vi "Write Array.vi"(8 "error in (no error)":errorcluster, 10 "Array":dbl[](array[numeric]), 11 "Doublo Array in":refnum<class "Doublo Array.lvclass">) -> (0 "error out":errorcluster, 3 "Doublo Array out":refnum<class "Doublo Array.lvclass">)   [LabVIEW 2020, in "Example Source.lvlib" / "Doublo Array.lvclass"]
uses:
  Doublo Array.lvclass
  Doublo Array.lvclass/Doublo Array.ctl
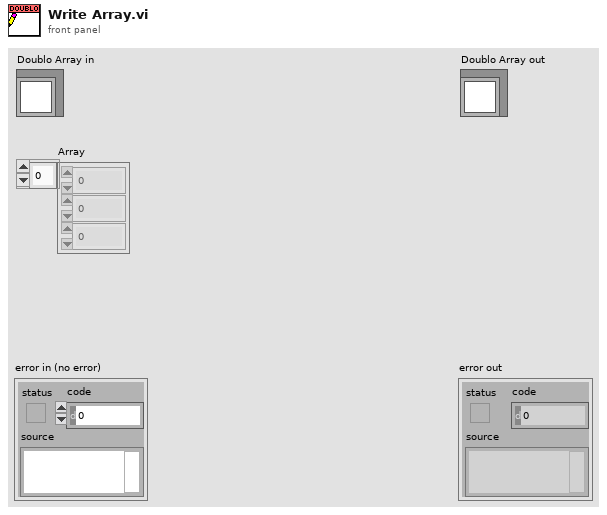
[diagram p1: front panel]
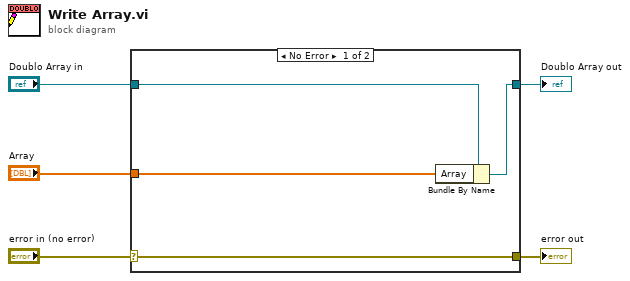
[diagram p0: block diagram]
diagram:
  n1 = case shown="No Error" "error in (no error)" {
    selector: "error in (no error)" -> [w9 w10]
    tunnel: [w9 w10] -> w4
    tunnel: [w7 w11] -> w2
    tunnel: "Doublo Array in" -> [w8 w11]
    tunnel: "Array" -> [w6 _]
    frame No Error {
      n2 = Bundle By Name(cluster=w8, "Array"=w6) -> (w7:refnum<class "Doublo Array.lvclass">)
    }
    frame Error {
    }
  }
  "error out" <- w4
  "Doublo Array out" <- w2
